vi "niRFSTS Sequence Flow Create Sequence.vi"(0 "Session Handle in":T1, 5 "Sequence Name":string, 11 "error in (no error)":errorcluster) -> (4 "Session Handle out":T1, 6 "New Sequence":refnum<k7>, 15 "error out":errorcluster)   [LabVIEW 2018, in "niRFSTS Sequence Flow.lvclass"]
uses:
  niRFSTS Sequence Flow.lvclass
  Typedefs/Session Handle.ctl
  niRFSTS Sequence Flow.lvclass/niRFSTS Sequence Flow.ctl
  Plugins/TestStand API Tools (TSAT).lvlibp/Sequence Actions/TSAT Sequence Actions.lvlib
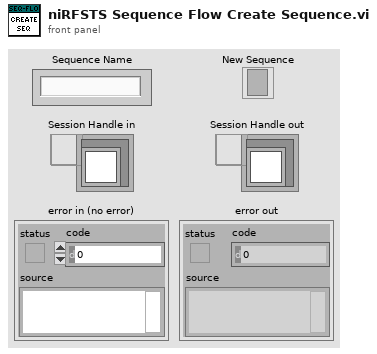
[diagram p1: front panel]
types:
  T1 = typedef "niRFSTS Sequence Flow.lvclass/Session Handle.ctl" = refnum<data-value>
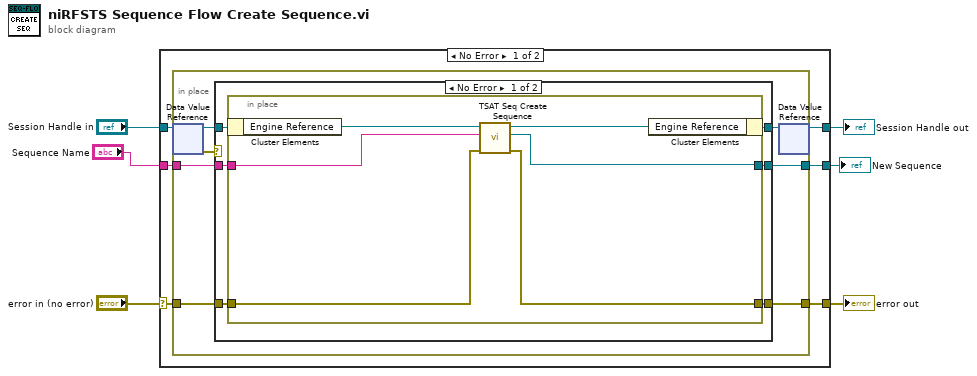
[diagram p0: block diagram]
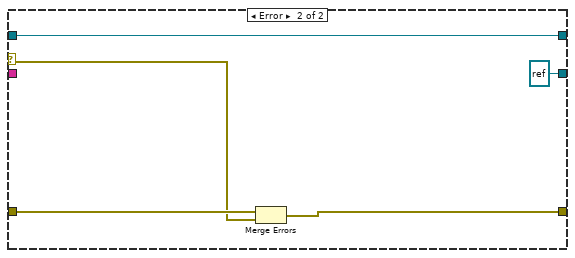
[diagram p2: hidden frame]
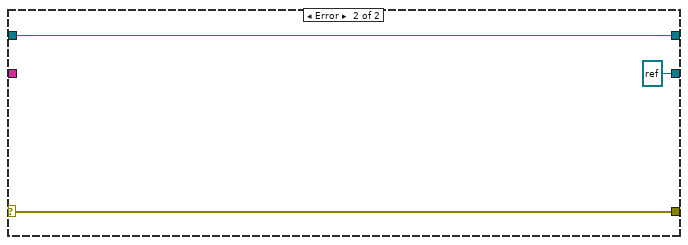
[diagram p3: hidden frame]
diagram:
  n1 = case shown="No Error" "error in (no error)" {
    selector: "error in (no error)" -> [w10 w38]
    tunnel: "Session Handle in" -> [w12 w39]
    tunnel: [w11 w39] -> w5
    tunnel: [w9 w38] -> w4
    tunnel: "Sequence Name" -> [w8 _]
    tunnel: [w7 refnum<k7> refnum ("Sequence Reference Out")] -> w1
    frame No Error {
      n2 = in-place {
        in-place-border: w10 -> [w15]
        in-place-border: [w18] -> w9
        in-place-border: w8 -> [w14]
        in-place-border: [w13] -> w7
        n3 = in-place-dvr #1(w12) -> (w19:refnum<class "niRFSTS Sequence Flow.lvclass">, w16:errorcluster)
        n4 = case shown="No Error" w16 {
          selector: w16 -> [_ w35]
          tunnel: w19 -> [w25 w33]
          tunnel: [w24 w34] -> w18
          tunnel: [w23 w33] -> w17
          tunnel: w15 -> [w22 w36]
          tunnel: w14 -> [w21 _]
          tunnel: [w20 refnum<k7> refnum ("Sequence Reference Out")] -> w13
          frame No Error {
            n5 = in-place {
              in-place-border: [w30] -> w24
              in-place-border: w22 -> [w31]
              in-place-border: w21 -> [w27]
              in-place-border: [w26] -> w20
              n6 = in-place-cluster #2(w25) -> ("Engine Reference"=w29:refnum<k7>)
              n7 = call "TSAT Seq Create Sequence.vi"("Error in"=w31, "Sequence Name"=w27, "Engine In"=w29) -> ("Error out"=w30:errorcluster, "Sequence Reference Out"=w26:refnum<k7>, "Engine Out"=w28:refnum<k7>)  [unwired: 6 in]
              n8 = in-place-cluster #2("Engine Reference"=w28) -> (w23:refnum<class "niRFSTS Sequence Flow.lvclass">)
            }
          }
          frame Error {
            n9 = Merge Errors(w36, w35) -> (w34:errorcluster)
          }
        }
        n10 = in-place-dvr #1(w17) -> (w11:T1)  [unwired: 1 out]
      }
    }
    frame Error {
    }
  }
  "Session Handle out" <- w5
  "error out" <- w4
  "New Sequence" <- w1
